vi "set_resolution.vi"(8 "error in (no error)":errorcluster, 9 "y":i32, 10 "x":i32, 11 "ImagingModeDL090130Frame in":refnum<class "ImagingModeDL090130Frame.lvclass">) -> (0 "error out":errorcluster, 3 "ImagingModeDL090130Frame out":refnum<class "ImagingModeDL090130Frame.lvclass">)   [LabVIEW 2010, in "ImagingModeDL090130Frame.lvclass"]
uses:
  ImagingModeDL090130Frame.lvclass
  ImagingModeDL090130Frame.lvclass/ImagingModeDL090130Frame.ctl
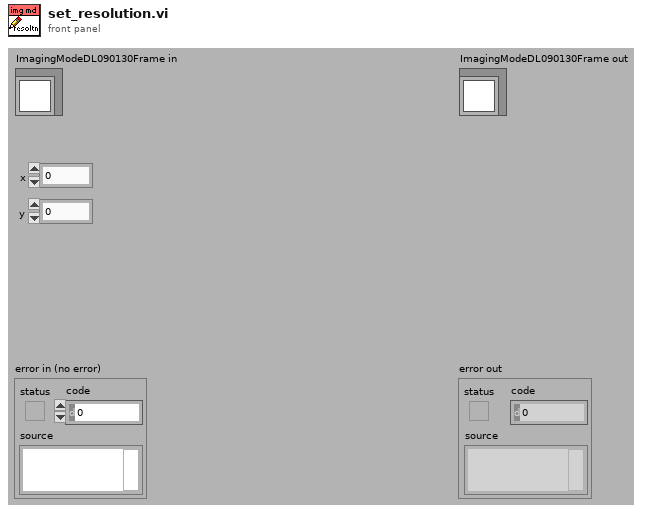
[diagram p1: front panel]
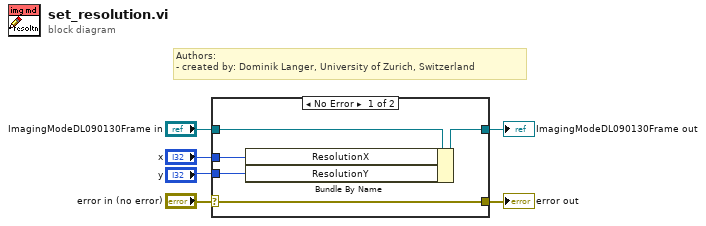
[diagram p0: block diagram]
diagram:
  # "Authors: \n- created by: Dominik Langer, University of Zurich, Switzerland"
  n1 = case shown="No Error" "error in (no error)" {
    selector: "error in (no error)" -> [w11 w13]
    tunnel: [w11 w13] -> w5
    tunnel: [w9 w12] -> w3
    tunnel: "ImagingModeDL090130Frame in" -> [w10 w12]
    tunnel: "y" -> [w8 _]
    tunnel: "x" -> [w7 _]
    frame No Error {
      n2 = Bundle By Name(cluster=w10, "ResolutionX"=w7, "ResolutionY"=w8) -> (w9:refnum<class "ImagingModeDL090130Frame.lvclass">)
    }
    frame Error {
    }
  }
  "error out" <- w5
  "ImagingModeDL090130Frame out" <- w3
